vi "Create Stub Files.vi"(8 "error in":errorcluster, 11 "Main Destination Path":path) -> (0 "error out":errorcluster)   [LabVIEW 2020]
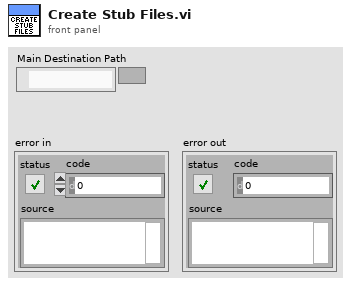
[diagram p1: front panel]
types:
  T1 = enum16{"open", "replace", "create", "open or create", "replace or create", "replace or create with confirmation"}
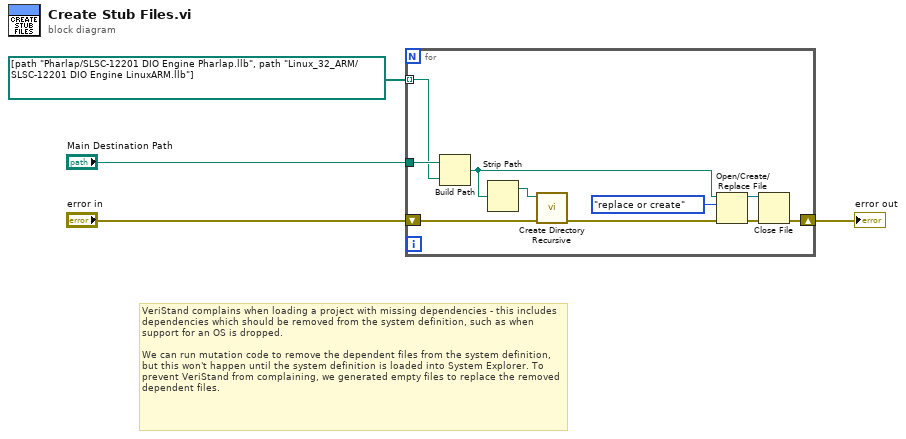
[diagram p0: block diagram]
diagram:
  # "VeriStand complains when loading a project with missing dependencies - this includes dependencies which should be removed from the system definition, such as when support for an OS is dropped.\n\nWe can run mutation code to remove the dependent files from the system definition, but this won't happen until the system definition is loaded into System Explorer. To prevent VeriStand from complaining, we generated empty files to replace the removed dependent files."
  n1 = for {
    tunnel: "Main Destination Path" -> [w14]
    tunnel: path[] [path "Pharlap/SLSC-12201 DIO Engine Pharlap.llb", path "Linux_32_ARM/SLSC-12201 DIO Engine LinuxARM.llb"] -> [w13] mode=indexing
    shift-right: [w9] -> w4
    shift-left: "error in" -> [w12]
    n2 = Build Path(base path=w14, name or relative path=w13) -> (appended path=w7:path)
    n3 = Strip Path(path=w7) -> (stripped path=w5:path)  [unwired: 1 out]
    n4 = call <vilib>:"Create Directory Recursive.vi"("error in (no error)"=w12, "directory"=w5) -> ("error out"=w6:errorcluster)  [unwired: 3 in, 2 out]
    n5 = Open/Create/Replace File(file path (use dialog)=w7, error in=w6, operation (0:open)=T1."replace or create") -> (refnum out=w8:refnum<file>, error out=w11:errorcluster)  [unwired: 3 in, 1 out]
    n6 = Close File(refnum=w8, error in=w11) -> (error out=w9:errorcluster)  [unwired: 1 out]
  }
  "error out" <- w4
